vi "Topo & GridSpectr_DriftCorrection_v11.vi"(6 "Internal use":string, 7 "Grid param":T1 {"height (m)" format="%#_6p"; "width (m)" format="%#_6p"; "center Y (m)" format="%#_6p"; "center X (m)" format="%#_6p"}, 8 "Error in (no error)":errorcluster, 9 "Points Y/Index Y":i32, 10 "Points X/Index X":i32, 11 "Method":enum16{"init", "run", "end"}(ring)=enum."end") -> (0 "Error out":errorcluster)   [LabVIEW 2014]
doc: "Example of a measurement VI to be used in the \"Experiments on a Grid\" tool as external VI.\n\nThis example measure the topography and spectroscopy data. The spectroscopy measurements are taken on a subgrid. The data are saved to a sxm and a binary file.\n\n- Nanonis Programming Interface -"
uses:
  <userlib>/Nanonis Prog Interface V5/Scan/Grid/GridPatternGet.vi
  <userlib>/Nanonis Prog Interface V5/Nanonis Prog Interface.lvlib
panel:
  in  "Lockin ON/OFF":bool
  in  "Correct Drift":bool
  in  "Email when finished":string="cornelius.krull@monash.edu"
  in  "STS z offset":dbl=1.15e-09 format="%#_6p"
  out "ETA":timestamp
  out "remaining":dbl format="%<%H:%M:%S>t"
  out "Progress":u8(slide) scale=0.0..100.0 scale format="%#.1g"
  out "total Points":i32
  in  "preSTS delay [ms]":u32=3
  in  "STS Bias":dbl=0.005 format="%#_6p"
  in  "Move Bias":dbl=-0.01 format="%#_6p"
  in  "Move Current":dbl=1.5e-11 format="%#_6p"
  in  "Imaging Bias":dbl=-0.01 format="%#_6p"
  in  "max applied Drift Correction":i32=20 min=1 max=100 step=1 format="%.0p"
  in  "Correlate":u16(ring) items=["first Frame", "successive Frames"]
  out "Topo Images taken":i32=14
  in  "Increment":i32=40
  in  "Threshold":i32=2 min=1 step=1
  in  "tip Speed (m/s)":sgl=1e-08 format="%.2p"
  out "X drift":i32
  out "Y drift":i32
  out "Last Drift detected":i32=40
  in  "MaxImagesBack":i32=40
  in  "Channel index (0-23)":u8=14
  in  "File name":string="single_mol_shortSTS"
  in  "STS Current":dbl=1.15e-09 format="%#_6p"
  in  "Imaging Current":dbl=1.5e-11 format="%#_6p"
  in  "zdrift \nDuration (s)":dbl
  in  "Correct z drift":bool
  out "Status":string="finishing"
  in  "Drift correction Pixels":i32=256 caption="Topo Pixels"
  out "Y Offset":dbl format="%#_6p"
  out "X Offset":dbl format="%#_6p"
  out "Points taken":dbl=14.0
  in  "Drift Correction every":i32=40
  in  "Y subgrid spacing":u16=1
  in  "X subgrid spacing":u16=1
  # "GRID points"
  # "Increase this if no Drift was detected for \na certain number of images"
  # "%"
  # "time (HH:MM:SS)"
  # "images back"
  # "% of image size"
  # "RUN smart tilt before starting the GRID"
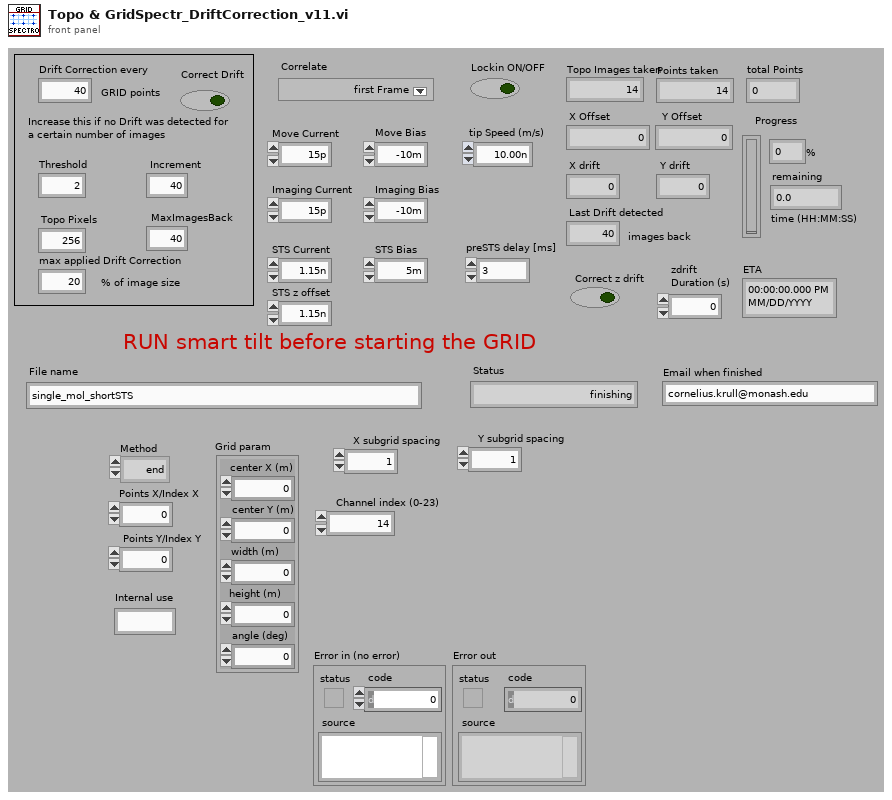
[diagram p1: front panel]
types:
  T1 = cluster{"center X (m)":sgl, "center Y (m)":sgl, "width (m)":sgl, "height (m)":sgl, "angle (deg)":sgl}
  T2 = cluster{"Drift correction Pixels":i32, "Imaging Current":dbl, "STS Current":dbl, "MaxImagesBack":i32, "tip Speed (m/s)":sgl, "Threshold":i32, "Increment":i32, "Correlate":u16, "max applied Drift Correction":i32, "Imaging Bias":dbl, "Move Current":dbl, "Move Bias":dbl, "STS Bias":dbl, "preSTS delay [ms]":u32, "STS z offset":dbl, "Correct Drift":bool, "Lockin ON/OFF":bool}
  T3 = cluster{"center X":sgl, "center Y":sgl, "angle":sgl, "width":sgl, "height":sgl, "# pixels":i32, "# lines":i32}
  T4 = cluster{"Name":string, "Calibration":sgl, "Offset":sgl, "Channel index":i32}[]
  T5 = cluster{"up/down":bool, "time/line":sgl, "start time":timestamp, "end time":timestamp}
  T6 = cluster{"Z averaging time (s)":sgl, "Z offset (m)":sgl, "Initial settling time (s)":sgl}
  T7 = cluster{"Max. slew rate (V/s)":sgl, "Settling time (s)":sgl, "Integration time (s)":sgl}
  T8 = cluster{"End settling time (s)":sgl, "Z control time (s)":sgl}
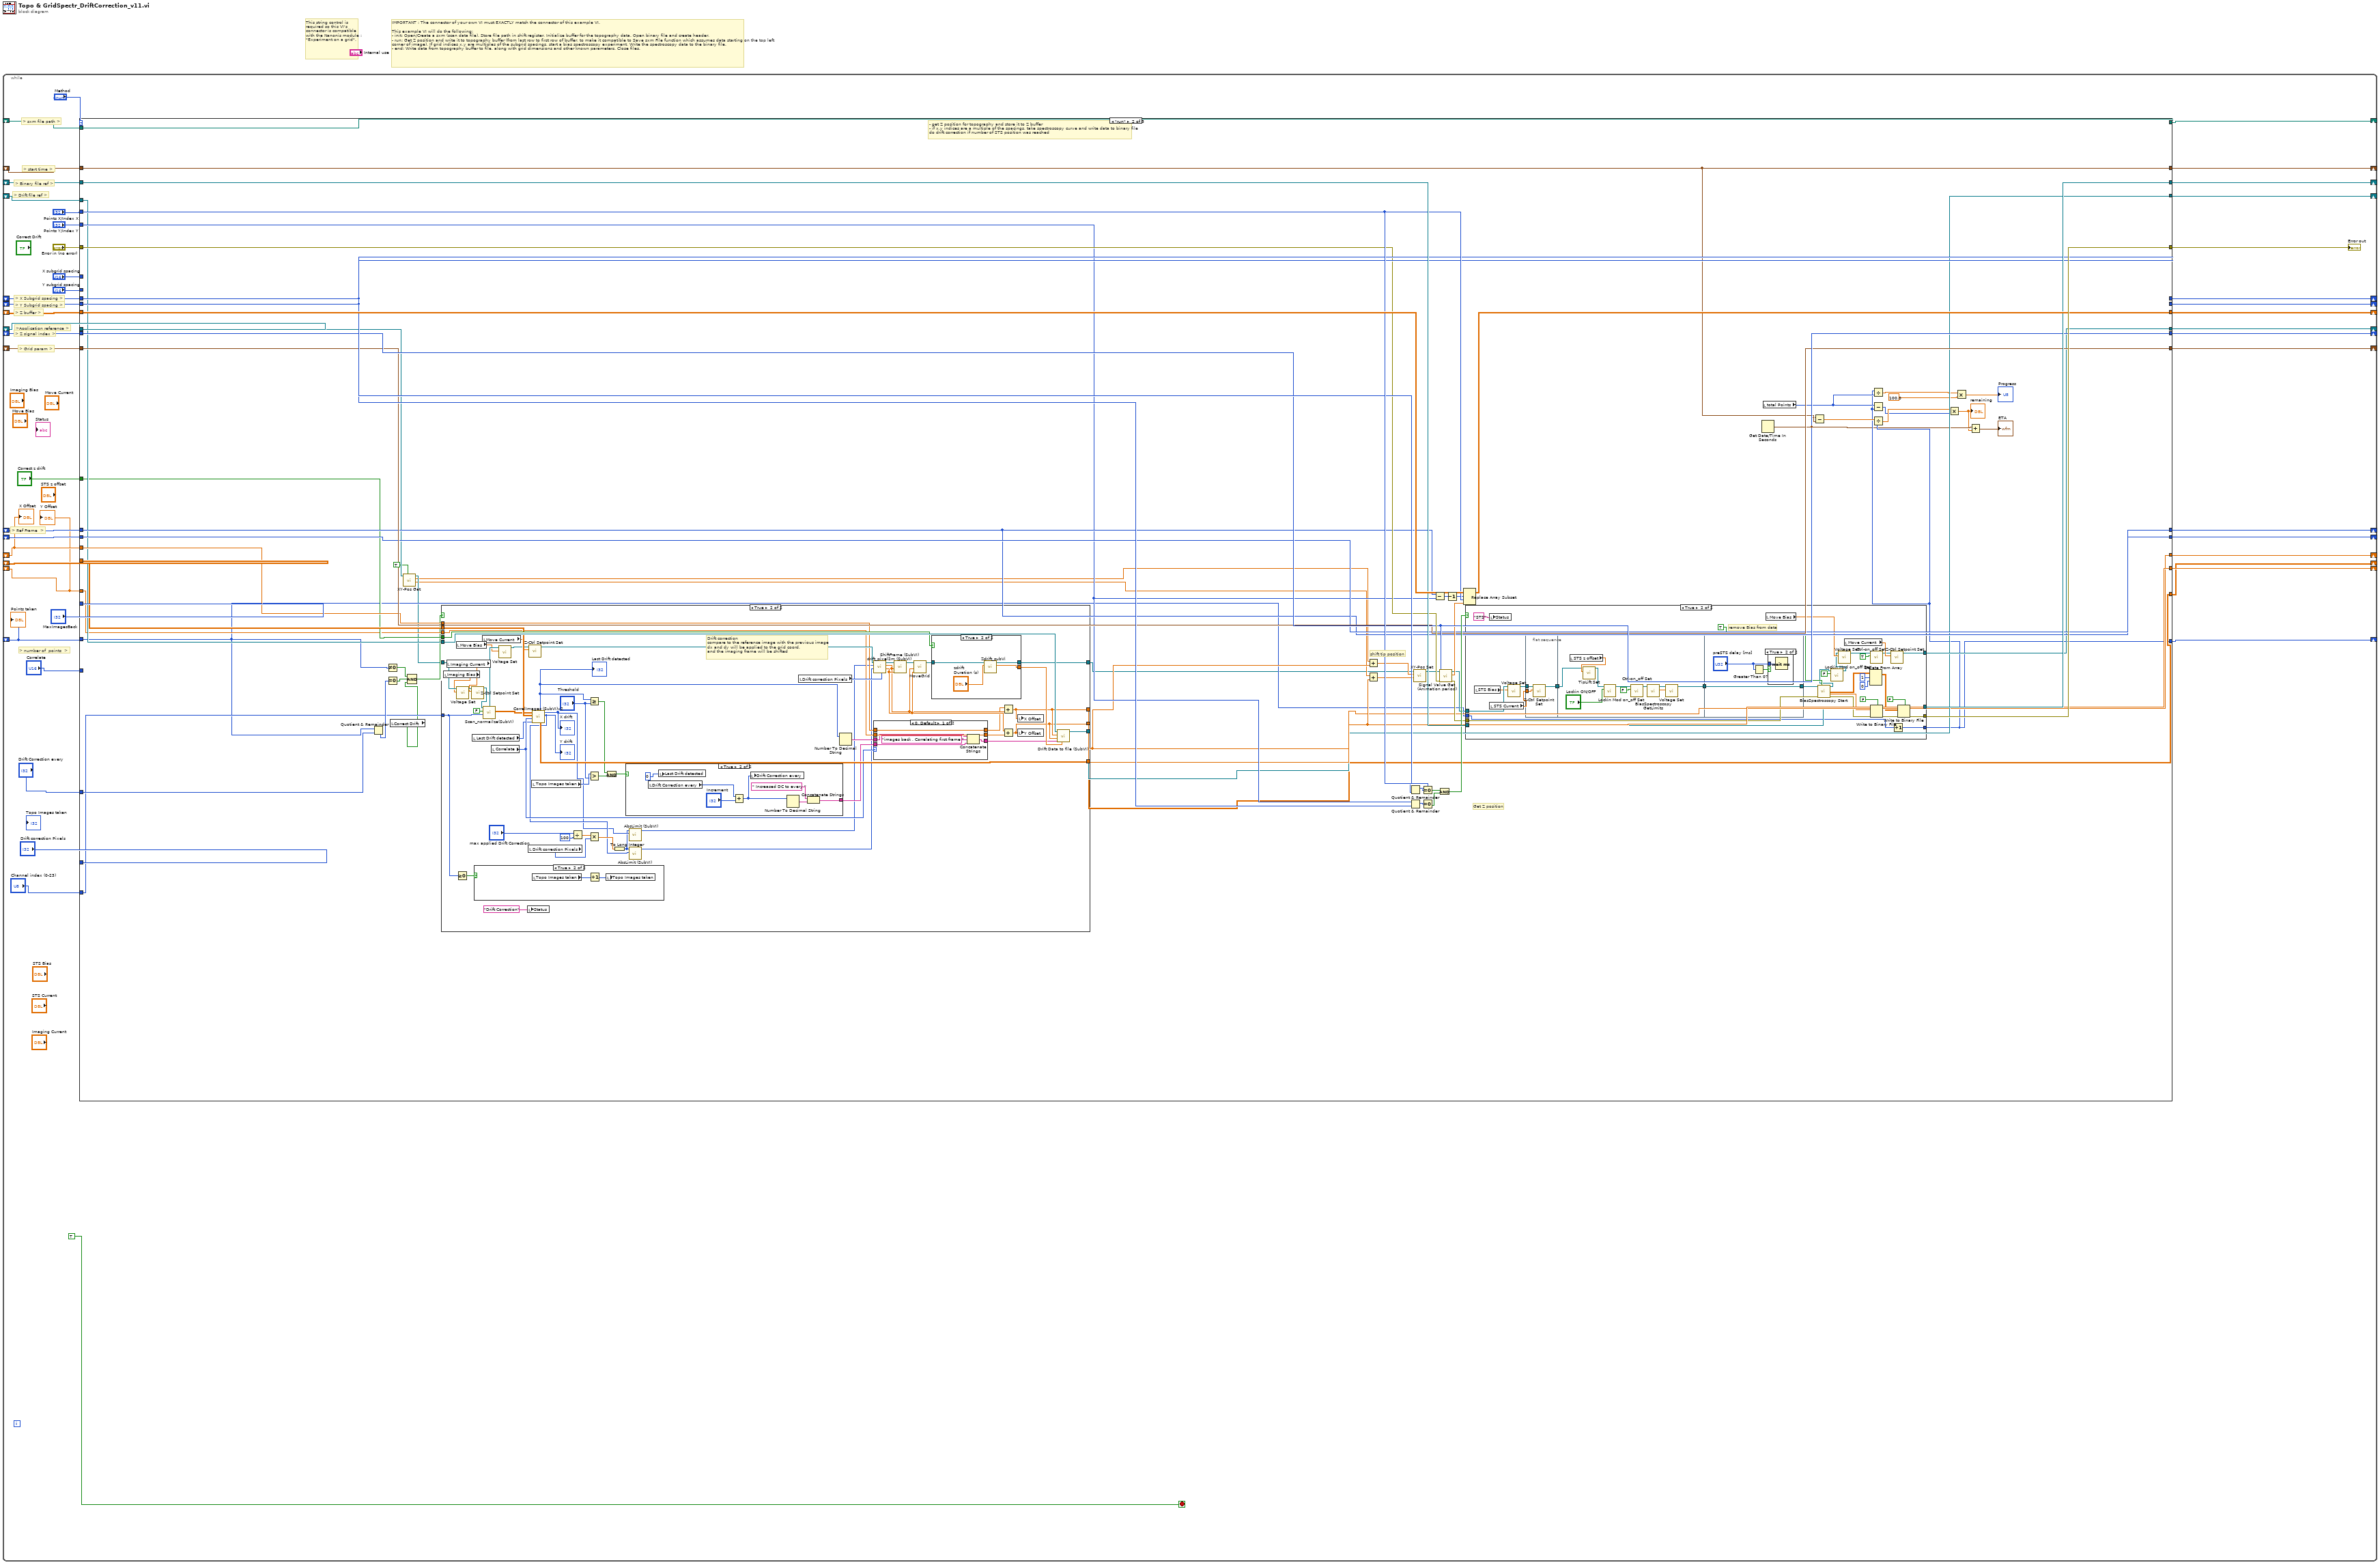
[diagram p0: block diagram]
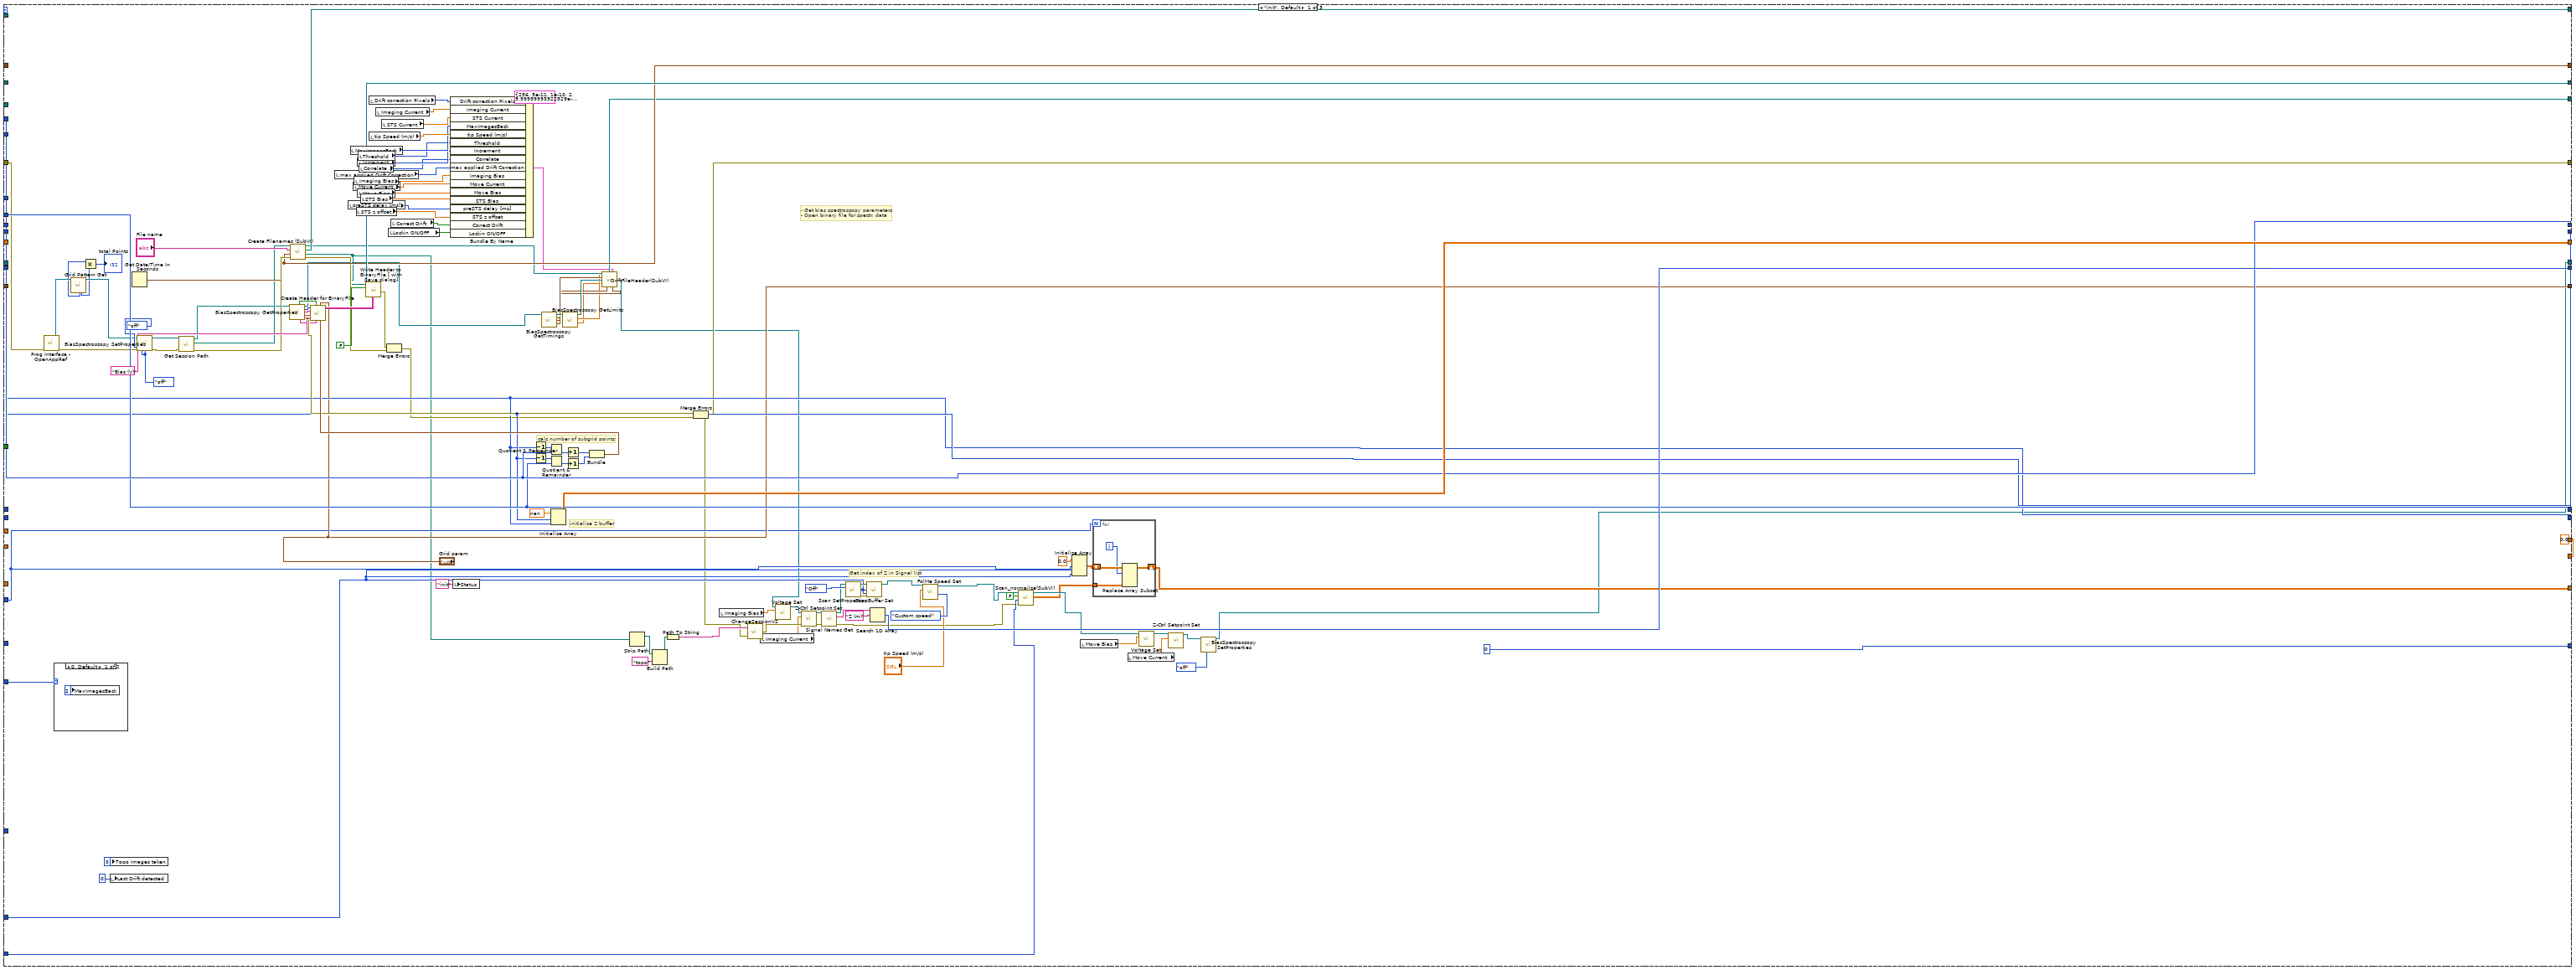
[diagram p2: hidden frame]
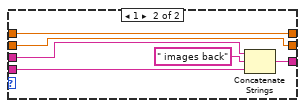
[diagram p5: hidden frame]
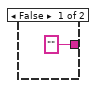
[diagram p7: hidden frame]
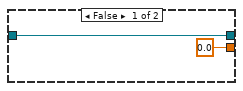
[diagram p8: hidden frame]
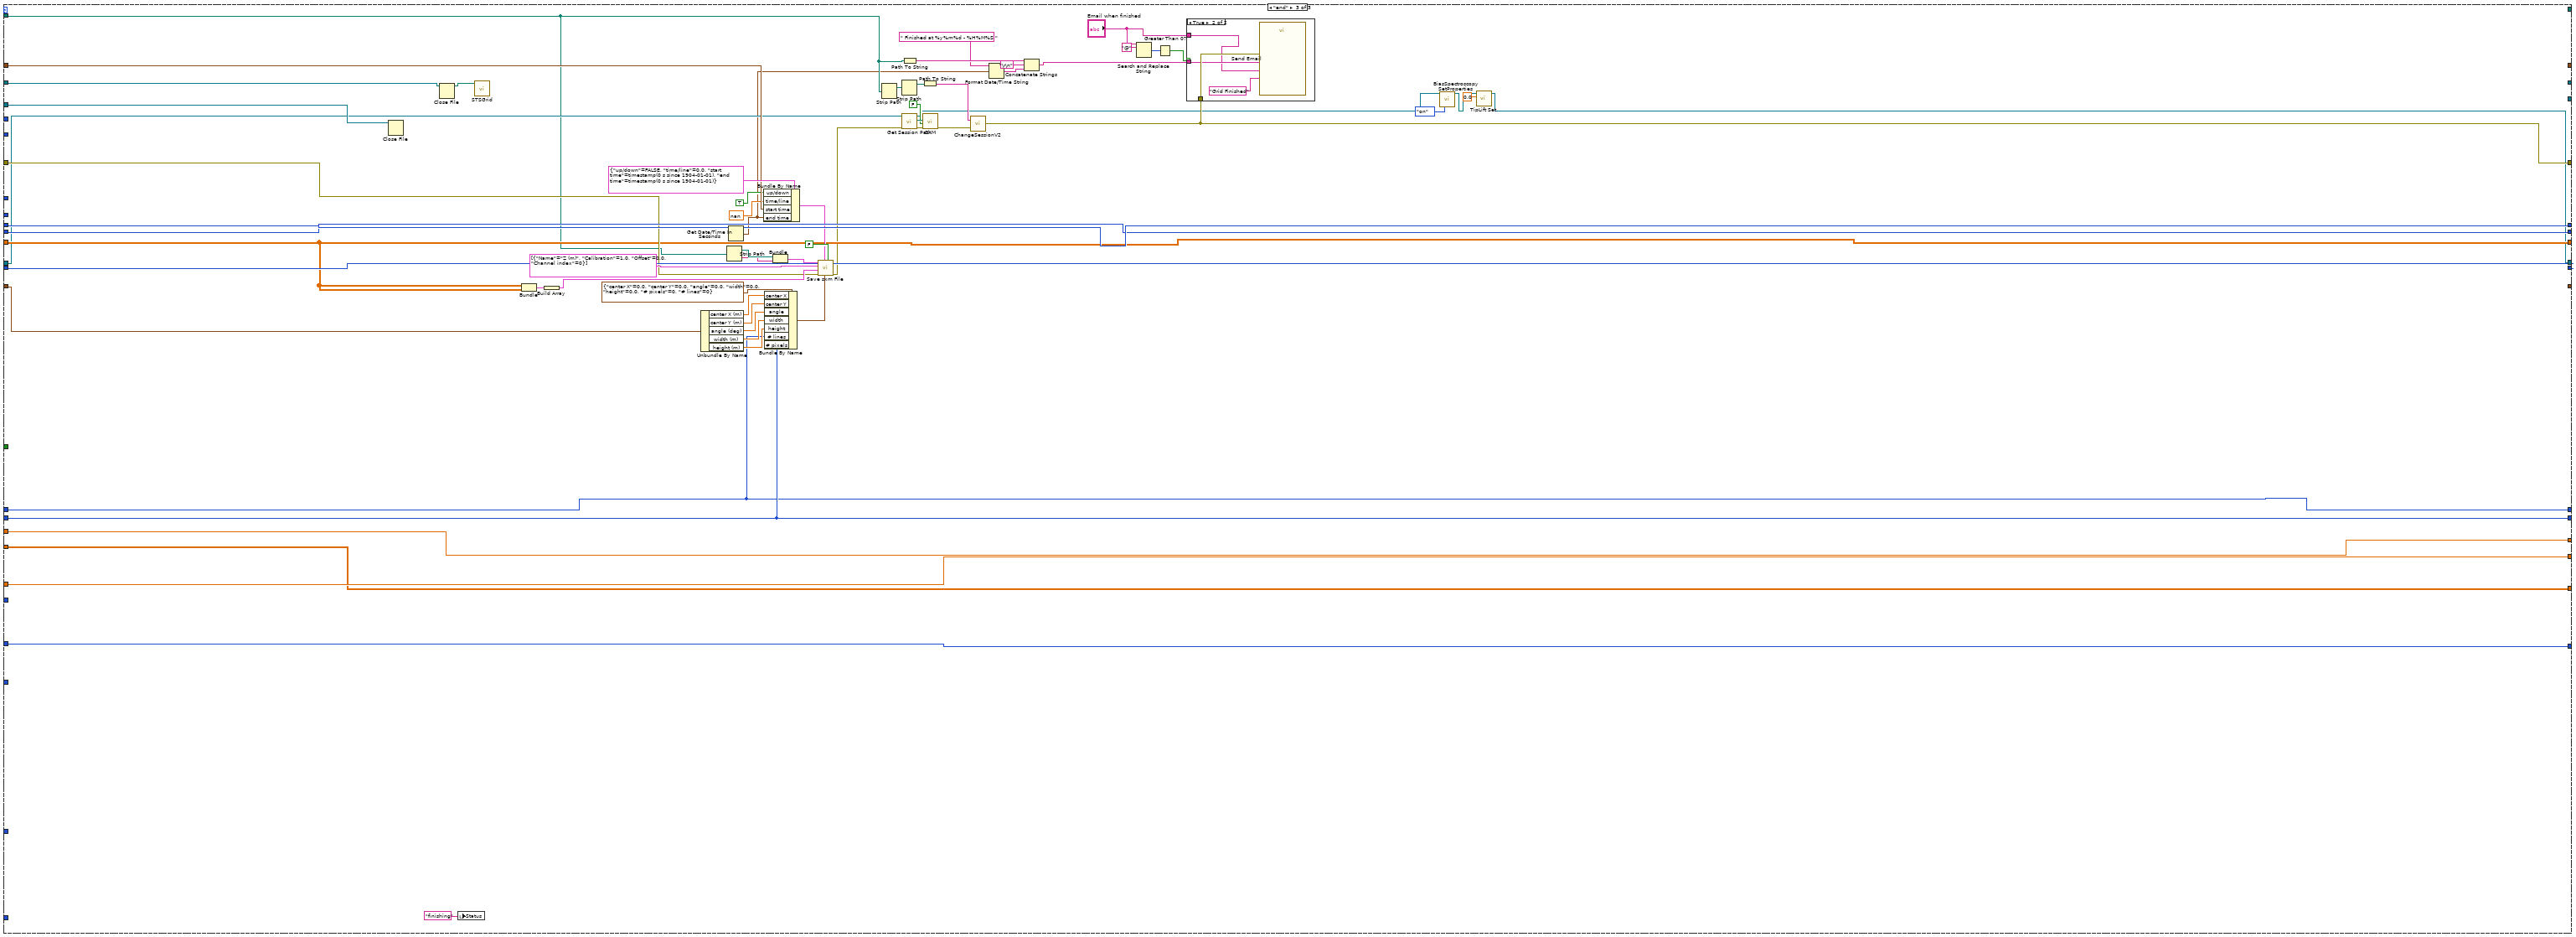
[diagram p11: hidden frame]
diagram:
  # "This string control is required so this VI's connector is compatible with the Nanonis module : \"Experiment on a grid\"."
  # "IMPORTANT : The connector of your own VI must EXACTLY match the connector of this example VI.\n\nThis example VI will do the following:\n- init: Open/Create a sxm (scan data file). Store file path in shift register. Initialize buffer for the topography data. Open binary file and create header.\n- run: Get Z position and write it to topography buffer (from last row to first row of buffer, to make it compatible to Save sxm File function which assumes data starting on the top left corner of image). If grid indices x,y are multiples of the subgrid spacings, start a bias spectroscopy experiment. Write the spectroscopy data to the binary file.\n- end: Write data from topography buffer to file, along with grid dimensions and other known parameters. Close files."
  n1 = while {
    shift-right: [w21] -> _
    shift-left: _ -> [w44]
    shift-right: [w39] -> _
    shift-left: _ -> [w38]
    shift-right: [w36] -> _
    shift-left: _ -> [w37]
    shift-right: [w35] -> _
    shift-left: _ -> [w34]
    shift-right: [w28] -> _
    shift-left: _ -> [w30]
    shift-right: [w29] -> _
    shift-left: _ -> [w31]
    shift-right: [w27] -> _
    shift-left: _ -> [w26]
    shift-right: [w25] -> _
    shift-left: _ -> [w24]
    shift-right: [w23] -> _
    shift-left: _ -> [w22]
    shift-right: [w20] -> _
    shift-left: _ -> [w19]
    shift-right: [w18] -> _
    shift-left: _ -> [w17]
    shift-right: [w16] -> _
    shift-left: _ -> [w9]
    shift-right: [w15] -> _
    shift-left: _ -> [w8]
    shift-right: [w14] -> _
    shift-left: _ -> [w11]
    shift-right: [w13] -> _
    shift-left: _ -> [w10]
    shift-right: [w6] -> _
    shift-left: _ -> [w5]
    stop <- TRUE stop-if-true
    # "> Drift file ref >"
    # "> number of  points  >"
    # "> Ref Frame  >"
    # "> Grid param >"
    # "> start time >"
    # ">Application reference >"
    # "> Y Subgrid spacing >"
    # "> X Subgrid spacing >"
    # "> Z signal index >"
    # "> Binary file ref >"
    # "> Z buffer >"
    # "> sxm file path >"
    n2 = case shown="\"run\"" "Method" {
      tunnel: [w127 w234 _] -> w21
      tunnel: w44 -> [_ w234 w393]
      tunnel: "Error in (no error)" -> [w129 w220 w424]
      tunnel: [w106 w233 w394] -> w42
      tunnel: "Points X/Index X" -> [w141 w228 _]
      tunnel: "Points Y/Index Y" -> [w142 w213 _]
      tunnel: [w165 w231 w413] -> w39
      tunnel: w38 -> [_ w232 w413]
      tunnel: w37 -> [_ w230 w406]
      tunnel: [w157 w229 _] -> w36
      tunnel: [w155 w218 w438] -> w35
      tunnel: w34 -> [_ w218 w438]
      tunnel: "X subgrid spacing" -> [w154 _ _]
      tunnel: "Y subgrid spacing" -> [w153 _ _]
      tunnel: w31 -> [_ w222 w437]
      tunnel: w30 -> [_ w221 w436]
      tunnel: [w154 w222 w437] -> w29
      tunnel: [w153 w221 w436] -> w28
      tunnel: [w84 w206 w379] -> w27
      tunnel: w26 -> [_ w189 w399]
      tunnel: ["Grid param" w216 _] -> w25
      tunnel: w24 -> [_ w216 w423]
      tunnel: [w126 w179 _] -> w23
      tunnel: w22 -> [_ w179 w431]
      tunnel: [w142 w214 w414] -> w20
      tunnel: w19 -> [_ w214 w414]
      tunnel: [w141 w215 w415] -> w18
      tunnel: w17 -> [_ w215 w415]
      tunnel: [w138 w196 w412] -> w16
      tunnel: [w138 w201 w410] -> w15
      tunnel: [w122 w195 w407] -> w14
      tunnel: [0 w177 w411] -> w13
      tunnel: w10 -> [_ w192 w411]
      tunnel: "Drift Correction every" -> [_ w209 _]
      tunnel: w11 -> [_ w200 w407]
      tunnel: w9 -> [_ w207 w412]
      tunnel: w8 -> [_ w193 w410]
      tunnel: "Drift correction Pixels" -> [w121 _ _]
      tunnel: [w79 w198 _] -> w6
      tunnel: w5 -> [_ w199 w408]
      tunnel: "Correct z drift" -> [_ w197 _]
      tunnel: "Channel index (0-23)" -> [w52 w194 _]
      tunnel: "MaxImagesBack" -> [w120 _ _]
      tunnel: "Correlate" -> [w98 _ _]
      frame "init", Default {
        w81 = enum16{"no change", "on", "off"}."off" ("Save dialog")
        w138 = 0.0
        # "- Get bias spectroscopy parameters\n- Open binary file for spectr. data"
        # "initialize Z buffer"
        # "calc number of subgrid points"
        # "Get index of Z in Signal list"
        n3 = call <userlib>:"Prog Interface - OpenAppRef.vi"("Error in (no error)"=w129) -> ("Error out"=w104:errorcluster, "Application reference"=w89:refnum<vi>)  [unwired: 5 in]
        n4 = case shown="0, Default" w98 {
          frame 0, Default {
            n5 = local write "MaxImagesBack"(2 ("StepsBack")) -> ()
          }
          frame 1 {
          }
        }
        n6 = call-poly <userlib>:"Grid Pattern Get.vi"("Application ref in"=w89) -> ("Points Y"=w86:i32, "Points X"=w87:i32, "Application ref out"=w88:refnum<vi>)  [unwired: 10 in, 6 out]
        n7 = Multiply(x=w86, y=w87) -> (x*y=→"total Points":i32)
        n8 = local write "Topo Images taken"(0 ("Images taken")) -> ()
        n9 = local write "Last Drift detected"(0 ("Last Drift detected")) -> ()
        n10 = Get Date/Time In Seconds() -> (seconds since 1Jan1904=w126:timestamp)
        n11 = call <userlib>:"BiasSpectroscopy SetProperties.vi"("Application ref in"=w88, "Autosave (no change)"=enum16{"no change", "on", "off"}."off", "Error in (no error)"=w104, "Z-Controller hold (no change)"=w81, "Save dialog"=w81) -> ("Application ref out"=w101:refnum<vi>, "Error out"=w100:errorcluster)  [unwired: 9 in]
        n12 = call <userlib>:"Get Session Path.vi"("error in (no error)"=w100, "Application ref in"=w101) -> ("error out"=w128:errorcluster, "Session path"=w112:path, "Application ref out"=w102:refnum<vi>)  [unwired: 7 in]
        n13 = call <userlib>:"BiasSpectroscopy GetProperties.vi"("Application ref in"=w102) -> ("Backward sweep"=w161:bool, "Application ref out"=w115:refnum<vi>, "Number of points"=w144:i32, "Channels"=w143:string[], "Parameters"=w159:string[], "Fixed parameters"=w146:string[], "Error out"=w158:errorcluster)  [unwired: 6 in, 2 out]
        n14 = call "Create Filenames (SubVI).vi"("error in (no error)"=w128, "seconds since 1Jan1904"=w126, "File name"="File name", "Session path"=w112) -> ("error out"=w116:errorcluster, "binFilePath"=w108:path, "topoFilePath"=w127:path, "Drift File out"=w80:refnum<file>)  [unwired: 4 in]
        n15 = local read "max applied Drift Correction"() -> (w60:i32)
        n16 = local read "preSTS delay [ms]"() -> (w55:u32)
        n17 = local read "MaxImagesBack"() -> (w64:i32)
        n18 = local read "Move Current"() -> (w58:dbl)
        n19 = local read "Imaging Bias"() -> (w59:dbl)
        n20 = local read "STS z offset"() -> (w54:dbl)
        n21 = local read "Increment"() -> (w62:i32)
        n22 = local read "Move Bias"() -> (w57:dbl)
        n23 = local read "Threshold"() -> (w63:i32)
        n24 = local read "Correlate"() -> (w61:u16)
        n25 = local read "STS Bias"() -> (w56:dbl)
        n26 = local read "Drift correction Pixels"() -> (w69:i32)
        n27 = local read "tip Speed (m/s)"() -> (w66:sgl)
        n28 = local read "Imaging Current"() -> (w68:dbl)
        n29 = local read "STS Current"() -> (w67:dbl)
        n30 = local read "Lockin ON/OFF"() -> (w65:bool)
        n31 = local read "Correct Drift"() -> (w53:bool)
        n32 = Bundle By Name(cluster=T2 {"Drift correction Pixels"=256, "Imaging Current"=5e-11, "STS Current"=1e-10, "MaxImagesBack"=2, "tip Speed (m/s)"=1e-08, "Threshold"=2, "Increment"=64, "Correlate"=0, "max applied Drift Correction"=20, "Imaging Bias"=-0.02, "Move Current"=1.5e-11, "Move Bias"=-0.02, "STS Bias"=0.1, "preSTS delay [ms]"=1000, "STS z offset"=-1.7e-10, "Correct Drift"=TRUE, "Lockin ON/OFF"=TRUE} ("Drift Correction"), "Drift correction Pixels"=w69, "Imaging Current"=w68, "STS Current"=w67, "MaxImagesBack"=w64, "tip Speed (m/s)"=w66, "Threshold"=w63, "Increment"=w62, "Correlate"=w61, "max applied Drift Correction"=w60, "Imaging Bias"=w59, "Move Current"=w58, "Move Bias"=w57, "STS Bias"=w56, "preSTS delay [ms]"=w55, "STS z offset"=w54, "Correct Drift"=w53, "Lockin ON/OFF"=w65) -> (w71:T2)
        n33 = local write "Status"("init" ("Status")) -> ()
        n34 = Decrement(x=w141) -> (x-1=w152:i32)
        n35 = Decrement(x=w142) -> (x-1=w151:i32)
        n36 = call <userlib>:"BiasSpectroscopy GetTimings.vi"("Application ref in"=w115) -> ("Application ref out"=w119:refnum<vi>, "Initialization"=w74:T6, "Sweep Timing"=w75:T7, "End of Sweep"=w76:T8)  [unwired: 10 in, 1 out]
        n37 = Quotient & Remainder(x=w152, y=w154) -> (floor(x/y)=w150:i32)  [unwired: 1 out]
        n38 = Quotient & Remainder(x=w151, y=w153) -> (floor(x/y)=w149:i32)  [unwired: 1 out]
        n39 = Initialize Array(sgl nan ("element"), w142, w141) -> (w165:sgl[][])
        n40 = call <userlib>:"BiasSpectroscopy GetLimits.vi"("Application ref in"=w119) -> ("End value (V)"=w72:sgl, "Start value (V)"=w73:sgl, "Application ref out"=w78:refnum<vi>)  [unwired: 5 in, 1 out]
        n41 = Increment(x=w150) -> (x+1=w148:i32)
        n42 = Increment(x=w149) -> (x+1=w147:i32)
        n43 = Bundle(w148, w147) -> (w160:cluster{i32, i32})  [unwired: 1 in]
        n44 = call <userlib>:"Create Header for BinaryFile.vi"("Grid points"=w160, "Grid param"="Grid param", "Fixed parameters"=w146, "Backward sweep"=w161, "Sweep signal"="Bias (V)" ("Sweep Signal"), "Parameters"=w159, "Channels"=w143, "Points per sweep"=w144) -> ("Header (fixed attributes)"=w163:string[][])  [unwired: 3 in]
        n45 = call <userlib>:"Write Header to BinaryFile [ with Save dialog].vi"("Fixed Attributes"=w163, "Show Dialog? (T)"=FALSE, "Filename"=w108) -> ("Error out"=w117:errorcluster, "File ref"=w157:refnum<file>)  [unwired: 5 in, 2 out]
        n46 = Merge Errors(w117, w116) -> (w118:errorcluster)
        n47 = call "DriftFileHeader(SubVI).vi"("Start value (V)"=w73, "Byte Stream File in"=w80, "Drift Correction"=w71, "End of Sweep"=w76, "Application ref in"=w78, "End value (V)"=w72, "Sweep Timing"=w75, "Initialization"=w74) -> ("Byte Stream File out"=w79:refnum<file>, "Application ref out"=w77:refnum<vi>)  [unwired: 6 in]
        n48 = Strip Path(path=w108) -> (stripped path=w111:path)  [unwired: 1 out]
        n49 = Build Path(base path=w111, name or relative path="topo") -> (appended path=w109:path)
        n50 = Path To String(path=w109) -> (string=w107:string)
        n51 = Merge Errors(w158, w118) -> (w106:errorcluster)
        n52 = local read "Imaging Bias"() -> (w91:dbl)
        n53 = call "ChangeSessionV2.vi"("error in (no error)"=w106, "Session"=w107) -> ("error out"=w105:errorcluster)
        n54 = local read "Imaging Current"() -> (w90:dbl)
        n55 = call <userlib>:"Voltage Set.vi"("Bias (V)"=w91, "Application ref in"=w77) -> ("Application ref out"=w94:refnum<vi>)  [unwired: 8 in, 1 out]
        n56 = call <userlib>:"Z-Ctrl Setpoint Set.vi"("error in (no error)"=w105, "Z Controller setpoint"=w90, "Application ref in"=w94) -> ("error out"=w130:errorcluster, "Application ref out"=w131:refnum<vi>)  [unwired: 7 in]
        n57 = call <userlib>:"Signal Names Get.vi"("error in (no error)"=w130, "Application ref in"=w131) -> ("error out"=w49:errorcluster, "Signals Names"=w145:string[], "Application ref out"=w134:refnum<vi>)  [unwired: 5 in]
        n58 = call <userlib>:"Scan SetProperties.vi"("Application ref in"=w134, "Continuous scan"=enum16{"No change", "On", "Off"}."Off") -> ("Application ref out"=w136:refnum<vi>, "Error out"=w135:errorcluster)  [unwired: 12 in]
        n59 = call <userlib>:"ScanBuffer Set.vi"("Application ref in"=w136, "Pixels"=w121, "Lines"=w121, "error in (no error)"=w135) -> ("Application ref out"=w96:refnum<vi>)  [unwired: 10 in, 1 out]
        n60 = Search 1D Array(1D array=w145, element="Z (m)") -> (index of element=w155:i32)  [unwired: 1 in]
        n61 = call <userlib>:"FolMe Speed Set.vi"("Speed Setting (Custom)"=enum32{"Scan speed", "Custom speed"}."Custom speed", "Speed (m/s)"="tip Speed (m/s)", "Application ref in"=w96) -> ("Application ref out"=w51:refnum<vi>)  [unwired: 5 in, 1 out]
        n62 = call "Scan_normailze(SubVI).vi"("error in (no error)"=w49, "Channel index (0-23)"=w52, "Normalization"=FALSE ("Boolean"), "Application in"=w51) -> ("Array"=w48:dbl[][], "Application out"=w50:refnum<vi>)  [unwired: 5 in, 1 out]
        n63 = Initialize Array(0.0 ("element"), w120, w121, w121) -> (w123:dbl[][][])
        n64 = local read "Move Bias"() -> (w93:dbl)
        n65 = for {
          N: w120 -> [_]
          tunnel: w48 -> [w169]
          shift-right: [w168] -> w122
          shift-left: w123 -> [w170]
          i -> [w167]
          n66 = Replace Array Subset(array=w170, new element=w169, index (dim 0)=w167) -> (w168:dbl[][][])  [unwired: 2 in]
        }
        n67 = local read "Move Current"() -> (w92:dbl)
        n68 = call <userlib>:"Voltage Set.vi"("Bias (V)"=w93, "Application ref in"=w50) -> ("Application ref out"=w95:refnum<vi>)  [unwired: 8 in, 1 out]
        n69 = call <userlib>:"Z-Ctrl Setpoint Set.vi"("Z Controller setpoint"=w92, "Application ref in"=w95) -> ("Application ref out"=w83:refnum<vi>)  [unwired: 8 in, 1 out]
        n70 = call <userlib>:"BiasSpectroscopy SetProperties.vi"("Application ref in"=w83, "Z-Controller hold (no change)"=enum16{"no change", "on", "off"}."off") -> ("Application ref out"=w84:refnum<vi>)  [unwired: 12 in, 1 out]
      }
      frame "run" {
        # "shift tip position"
        # "Get Z position"
        # "- get Z position for topography and store it to Z buffer\n- if x,y indices are a multiple of the spacings, take spectroscopy curve and write data to binary file\ndo drift correction if number of STS position was reached"
        n71 = Quotient & Remainder(x=w192, y=w209) -> (x-y*floor(x/y)=w210:i32)  [unwired: 1 out]
        n72 = Not Equal To 0?(x=w192) -> (x != 0?=w190:bool)
        n73 = Equal To 0?(x=w210) -> (x = 0?=w208:bool)
        n74 = local read "Correct Drift"() -> (w171:bool)
        n75 = call <userlib>:"XY-Pos Get.vi"("Wait for newest data (F=False)"=TRUE, "Application ref in"=w189) -> ("Y (m)"=w185:sgl, "X (m)"=w186:sgl, "Application ref out"=w188:refnum<vi>)  [unwired: 5 in, 1 out]
        n76 = Compound Arithmetic op=AND(w190, w208, w171) -> (w191:bool)
        n77 = case shown="True" w191 {
          tunnel: w188 -> [w239 w248]
          tunnel: [w239 w290] -> w184
          tunnel: w200 -> [w236 w285]
          tunnel: [w238 w288] -> w196
          tunnel: [w237 w287] -> w201
          tunnel: w207 -> [w238 w264]
          tunnel: w193 -> [w237 w262]
          tunnel: [w236 w281] -> w195
          tunnel: w199 -> [w235 w293]
          tunnel: [w235 w292] -> w198
          tunnel: w197 -> [_ w289]
          tunnel: w194 -> [_ w268]
          frame False {
          }
          frame True {
            # "Drift correction \ncompare to the reference image with the previous image \ndx and dy will be applied to the grid coord, \nand the imaging frame will be shifted"
            n78 = local read "Imaging Bias"() -> (w246:dbl)
            n79 = local read "Imaging Current"() -> (w245:dbl)
            n80 = local read "Move Bias"() -> (w242:dbl)
            n81 = Greater Or Equal To 0?(x=w268) -> (x >= 0?=w267:bool)
            n82 = call <userlib>:"Voltage Set.vi"("Bias (V)"=w246, "Application ref in"=w248) -> ("Application ref out"=w247:refnum<vi>)  [unwired: 8 in, 1 out]
            n83 = call <userlib>:"Z-Ctrl Setpoint Set.vi"("Z Controller setpoint"=w245, "Application ref in"=w247) -> ("Application ref out"=w286:refnum<vi>)  [unwired: 8 in, 1 out]
            n84 = local read "Last Drift detected"() -> (w259:i32)
            n85 = case shown="True" w267 {
              frame False {
              }
              frame True {
                n86 = local read "Topo Images taken"() -> (w308:i32)
                n87 = Increment(x=w308) -> (x+1=w307:i32)
                n88 = local write "Topo Images taken"(w307) -> ()
              }
            }
            n89 = local read "Move Current"() -> (w241:dbl)
            n90 = call "Scan_normailze(SubVI).vi"("Channel index (0-23)"=w268, "Normalization"=FALSE ("Boolean"), "Application in"=w286) -> ("Array"=w282:dbl[][], "Application out"=w243:refnum<vi>)  [unwired: 6 in, 1 out]
            n91 = local read "Correlate"() -> (w265:u16)
            n92 = call <userlib>:"Voltage Set.vi"("Bias (V)"=w242, "Application ref in"=w243) -> ("Application ref out"=w244:refnum<vi>)  [unwired: 8 in, 1 out]
            n93 = local write "Status"("Drift Correction" ("Status")) -> ()
            n94 = local read "Drift correction Pixels"() -> (w256:i32)
            n95 = call <userlib>:"Z-Ctrl Setpoint Set.vi"("Z Controller setpoint"=w241, "Application ref in"=w244) -> ("Application ref out"=w277:refnum<vi>)  [unwired: 8 in, 1 out]
            n96 = local read "Topo Images taken"() -> (w270:i32)
            n97 = call "CorrelImages (SubVI)v2.vi"("last drift detected"=w259, "Correlate"=w265, "Ref Array"=w285, "New Image"=w282) -> ("Y drift"=w253:i32, "X drift"=w250:i32, "Ref Array out"=w281:dbl[][][], "Queue Steps"=w266:i32)  [unwired: 4 in]
            "X drift" <- w250
            "Y drift" <- w253
            "Last Drift detected" <- w266
            n98 = Divide(x="max applied Drift Correction", y=100) -> (x/y=w255:dbl)
            n99 = Greater Or Equal?(x=w266, y="Threshold") -> (x >= y?=w272:bool)
            n100 = Greater?(x=w270, y="Threshold") -> (0:w269:bool)
            n101 = Multiply(x=w255, y=w256) -> (x*y=w257:dbl)
            n102 = And(x=w272, y=w269) -> (x .and. y?=w271:bool)
            n103 = To Long Integer(number=w257) -> (32bit integer=w249:i32)
            n104 = case shown="True" w271 {
              tunnel: ["" w312] -> w273
              frame False {
              }
              frame True {
                n105 = local read "Drift Correction every"() -> (w311:i32)
                n106 = local write "Last Drift detected"(0 ("Last Drift detected")) -> ()
                n107 = Add(x=w311, y="Increment") -> (x+y=w315:i32)
                n108 = local write "Drift Correction every"(w315) -> ()
                n109 = Number To Decimal String(number=w315) -> (decimal integer string=w314:string)  [unwired: 1 in]
                n110 = Concatenate Strings(" Increased DC to every " ("string"), w314) -> (w312:string)
              }
            }
            n111 = call "AbsLimit (SubVI).vi"("in"=w250, "Abslimt"=w249) -> ("Numeric out"=w252:i32)  [unwired: 9 in]
            n112 = call "AbsLimit (SubVI).vi"("in"=w253, "Abslimt"=w249) -> ("Numeric out"=w251:i32)  [unwired: 9 in]
            n113 = local read "Drift correction Pixels"() -> (w278:i32)
            n114 = Number To Decimal String(number=w266) -> (decimal integer string=w284:string)  [unwired: 1 in]
            n115 = call "drift_pixel2m (SubVI).vi"("Application in"=w277, "X drift"=w252, "Y drift"=w251, "Drift correction Pixels"=w278) -> ("Application out"=w276:refnum<vi>, "x drift"=w274:sgl, "y drift"=w275:sgl)  [unwired: 2 in, 1 out]
            n116 = case shown="0, Default" w265 {
              tunnel: w284 -> [w295 w306]
              tunnel: [w300 w305] -> w283
              tunnel: w273 -> [w298 w303]
              tunnel: w264 -> [w296 w302]
              tunnel: [w296 w302] -> w263
              tunnel: w262 -> [w297 w301]
              tunnel: [w297 w301] -> w261
              frame 0, Default {
                n117 = Concatenate Strings(w295, "images back , Correlating first frame " ("string"), w298) -> (w300:string)
              }
              frame 1 {
                n118 = Concatenate Strings(w306, " images back" ("string"), w303) -> (w305:string)
              }
            }
            n119 = call "ShiftFrame (SubVI).vi"("Y shift"=w275, "X shift"=w274, "Application in"=w276) -> ("Application out"=w280:refnum<vi>)  [unwired: 8 in]
            n120 = call "MoveGrid.vi"("y"=w275, "x"=w274, "Application ref in"=w280) -> ("Application ref out"=w279:refnum<vi>)  [unwired: 7 in, 1 out]
            n121 = case shown="True" w289 {
              tunnel: [0.0 ("z drift") w322] -> w291
              tunnel: w279 -> [w317 w321]
              tunnel: [w317 w320] -> w290
              frame False {
              }
              frame True {
                n122 = call "Zdrift_subVi.vi"("Duration"="zdrift \nDuration (s)", "Application in"=w321) -> ("z drift"=w322:dbl, "Application out"=w320:refnum<vi>)  [unwired: 7 in, 1 out]
              }
            }
            n123 = Add(x=w263, y=w274) -> (x+y=w288:dbl)
            n124 = Add(x=w275, y=w261) -> (x+y=w287:dbl)
            n125 = local write "X Offset"(w288) -> ()
            n126 = local write "Y Offset"(w287) -> ()
            n127 = call "Drift Data to file (SubVI).vi"("z drift"=w291, "Comment"=w283, "y Drift"=w287, "X drift"=w288, "Byte Stream File in"=w293) -> ("Byte Stream File out"=w292:refnum<file>)  [unwired: 6 in]
          }
        }
        n128 = Add(x=w186, y=w196) -> (x+y=w203:dbl)
        n129 = Add(x=w185, y=w201) -> (x+y=w202:dbl)
        n130 = Quotient & Remainder(x=w228, y=w222) -> (x-y*floor(x/y)=w227:i32)  [unwired: 1 out]
        n131 = Quotient & Remainder(x=w213, y=w221) -> (x-y*floor(x/y)=w226:i32)  [unwired: 1 out]
        n132 = call <userlib>:"XY-Pos Set.vi"("Y (m)"=w202, "X (m)"=w203, "Application ref in"=w184) -> ("Application ref out"=w204:refnum<vi>)  [unwired: 5 in, 1 out]
        n133 = Equal To 0?(x=w227) -> (x = 0?=w225:bool)
        n134 = Equal To 0?(x=w226) -> (x = 0?=w224:bool)
        n135 = Subtract(x=w214, y=w213) -> (x-y=w212:i32)
        n136 = And(x=w225, y=w224) -> (x .and. y?=w223:bool)
        n137 = call <userlib>:"Signal Value Get (Animation period).vi"("error in (no error)"=w220, "Signal index (0-47)"=w218, "Application ref in"=w204) -> ("error out"=w219:errorcluster, "Signal value"=w217:sgl, "Application ref out"=w205:refnum<vi>)  [unwired: 5 in]
        n138 = Decrement(x=w212) -> (x-1=w211:i32)
        n139 = Replace Array Subset(array=w232, new element=w217, index (row)=w211, index (col)=w228) -> (w231:sgl[][])
        n140 = case shown="True" w223 {
          tunnel: [w325 w346] -> w233
          tunnel: w230 -> [w326 w360]
          tunnel: [w326 w358] -> w229
          tunnel: w219 -> [w325 w357]
          tunnel: w205 -> [w324 w342]
          tunnel: [w324 w337] -> w206
          tunnel: [w323 w344] -> w177
          tunnel: w192 -> [w323 w345]
          frame False {
            # "Point indices aren't multiple of subgrid spacing\n=> no spectroscopy at this point"
          }
          frame True {
            # "remove Bias from data"
            n141 = local read "STS Bias"() -> (w339:dbl)
            n142 = local write "Status"("STS" ("Status")) -> ()
            n143 = local read "STS Current"() -> (w338:dbl)
            n144 = call <userlib>:"Voltage Set.vi"("Bias (V)"=w339, "Application ref in"=w342) -> ("Application ref out"=w341:refnum<vi>)  [unwired: 8 in, 1 out]
            n145 = flat-sequence {
              tunnel: w341 -> [w363]
              tunnel: w338 -> [w361]
              tunnel: [w362] -> w334
              tunnel: w334 -> [w366]
              tunnel: [w364] -> w333
              tunnel: [w376] -> w340
              tunnel: w333 -> [w376]
              frame #0 {
                n146 = call <userlib>:"Z-Ctrl Setpoint Set.vi"("Z Controller setpoint"=w361, "Application ref in"=w363) -> ("Application ref out"=w362:refnum<vi>)  [unwired: 8 in, 1 out]
              }
              frame #1 {
                n147 = local read "STS z offset"() -> (w369:dbl)
                n148 = call <userlib>:"TipLift Set.vi"("TipLift (m)"=w369, "Application ref in"=w366) -> ("Application ref out"=w365:refnum<vi>)  [unwired: 8 in, 1 out]
                n149 = call <userlib>:"Lockin Mod on_off Set.vi"("Lockin ON/OFF"="Lockin ON/OFF", "Application ref in"=w365) -> ("Application ref out"=w368:refnum<vi>)  [unwired: 8 in, 1 out]
                n150 = call <userlib>:"Ctrl-on_off Set.vi"("Z Controller ON/OFF"=FALSE, "Application ref in"=w368) -> ("Application ref out"=w371:refnum<vi>)  [unwired: 8 in, 1 out]
                n151 = call <userlib>:"BiasSpectroscopy GetLimits.vi"("Application ref in"=w371) -> ("Start value (V)"=w370:sgl, "Application ref out"=w372:refnum<vi>)  [unwired: 5 in, 2 out]
                n152 = call <userlib>:"Voltage Set.vi"("Bias (V)"=w370, "Application ref in"=w372) -> ("Application ref out"=w364:refnum<vi>)  [unwired: 8 in, 1 out]
              }
              frame #2 {
                n153 = Greater Than 0?(x="preSTS delay [ms]") -> (x > 0?=w374:bool)
                n154 = case shown="True" w374 {
                  tunnel: "preSTS delay [ms]" -> [_ w377]
                  frame False {
                  }
                  frame True {
                    n155 = Wait (ms)(milliseconds to wait=w377) -> ()  [unwired: 1 out]
                  }
                }
              }
            }
            n156 = local read "Move Bias"() -> (w336:dbl)
            n157 = call <userlib>:"BiasSpectroscopy Start.vi"("Application ref in"=w340, "Get data (F)"=TRUE ("Get Data (F)"), "Error in (no error)"=w357) -> ("Application ref out"=w329:refnum<vi>, "Data"=w356:sgl[][], "Parameters"=w355:sgl[], "Error out"=w348:errorcluster)  [unwired: 8 in, 1 out]
            n158 = call <userlib>:"Lockin Mod on_off Set.vi"("Lockin ON/OFF"=FALSE, "Application ref in"=w329) -> ("Application ref out"=w328:refnum<vi>)  [unwired: 8 in, 1 out]
            n159 = call <userlib>:"Voltage Set.vi"("Bias (V)"=w336, "Application ref in"=w328) -> ("Application ref out"=w331:refnum<vi>)  [unwired: 8 in, 1 out]
            n160 = local read "Move Current"() -> (w335:dbl)
            n161 = Delete From Array(array=w356, length=1, index (row)=0 ("index")) -> (array with subset deleted=w354:sgl[][])  [unwired: 1 in, 1 out]
            n162 = call <userlib>:"Ctrl-on_off Set.vi"("Z Controller ON/OFF"=TRUE, "Application ref in"=w331) -> ("Application ref out"=w330:refnum<vi>)  [unwired: 8 in, 1 out]
            n163 = Write to Binary File(file (use dialog)=w360, data=w355, error in=w348, 5:FALSE ("prepend array or string size? (T)")) -> (refnum out=w359:refnum<file>, error out=w347:errorcluster)  [unwired: 2 in, 1 out]
            n164 = call <userlib>:"Z-Ctrl Setpoint Set.vi"("Z Controller setpoint"=w335, "Application ref in"=w330) -> ("Application ref out"=w337:refnum<vi>)  [unwired: 8 in, 1 out]
            n165 = Increment(x=w345) -> (x+1=w344:i32)
            n166 = Write to Binary File(file (use dialog)=w359, data=w354, error in=w347, 5:FALSE ("prepend array or string size? (T)")) -> (refnum out=w358:refnum<file>, error out=w346:errorcluster)  [unwired: 2 in, 1 out]
          }
        }
        n167 = Get Date/Time In Seconds() -> (seconds since 1Jan1904=w174:timestamp)
        n168 = local read "total Points"() -> (w180:i32)
        n169 = Subtract(x=w174, y=w179) -> (x-y=w178:dbl)
        n170 = Divide(x=w177, y=w180) -> (x/y=w183:dbl)
        n171 = Subtract(x=w180, y=w177) -> (x-y=w175:i32)
        n172 = Divide(x=w178, y=w177) -> (x/y=w176:dbl)
        n173 = Multiply(x=w176, y=w175) -> (x*y=w173:dbl)
        "remaining" <- w173
        n174 = Multiply(x=w183, y=100.0) -> (x*y=→"Progress":dbl)
        n175 = Add(x=w174, y=w173) -> (x+y=→"ETA":timestamp)
      }
      frame "end" {
        n176 = Close File(refnum=w408) -> ()  [unwired: 1 in, 2 out]
        n177 = Close File(refnum=w406) -> (path=w405:path)  [unwired: 1 in, 1 out]
        n178 = local write "Status"("finishing" ("Status")) -> ()
        n179 = call "STSGrid.vi"("Binary Spectroscopy File"=w405) -> ()  [unwired: 11 in]
        n180 = Bundle(w413, w413) -> (w435:cluster{sgl[][], sgl[][]})  [unwired: 1 in]
        n181 = Build Array(w435) -> (w434:cluster{sgl[][], sgl[][]}[])
        n182 = Unbundle By Name(w423) -> ("center X (m)"=w421:sgl, "center Y (m)"=w420:sgl, "angle (deg)"=w419:sgl, "width (m)"=w418:sgl, "height (m)"=w417:sgl)
        n183 = Strip Path(path=w393) -> (stripped path=w427:path, name=w426:string)
        n184 = Get Date/Time In Seconds() -> (seconds since 1Jan1904=w389:timestamp)
        n185 = Bundle By Name(cluster=T5 {"up/down"=FALSE, "time/line"=0.0, "start time"=timestamp(0 s since 1904-01-01), "end time"=timestamp(0 s since 1904-01-01)} ("Scan param"), "up/down"=TRUE, "time/line"=sgl nan ("input 7"), "start time"=w431, "end time"=w389) -> (w430:T5)
        n186 = Bundle By Name(cluster=T3 {"center X"=0.0, "center Y"=0.0, "angle"=0.0, "width"=0.0, "height"=0.0, "# pixels"=0, "# lines"=0} ("Scanfield"), "center X"=w421, "center Y"=w420, "angle"=w419, "width"=w418, "height"=w417, "# lines"=w414, "# pixels"=w415) -> (w416:T3)
        n187 = Bundle("stripped path"=w427, "name"=w426) -> (w425:cluster{"stripped path":path, "name":string})  [unwired: 1 in]
        n188 = call <userlib>:"Save sxm File.vi"("Auto file naming? (T)"=FALSE, "Scanfield"=w416, "Scan param"=w430, "error in (no error)"=w424, "Channels data"=w434, "Channels config"=T4 [{"Name"="Z (m)", "Calibration"=1.0, "Offset"=0.0, "Channel index"=0}], "Filename control"=w425) -> ("error out"=w400:errorcluster)  [unwired: 2 in, 2 out]
        n189 = Strip Path(path=w393) -> (stripped path=w404:path)  [unwired: 1 out]
        n190 = Strip Path(path=w404) -> (stripped path=w403:path)  [unwired: 1 out]
        n191 = call <userlib>:"Get Session Path.vi"("error in (no error)"=w400, "Application ref in"=w399) -> ("error out"=w396:errorcluster, "Session path"=w398:path, "Application ref out"=w382:refnum<vi>)  [unwired: 7 in]
        n192 = Path To String(path=w393) -> (string=w392:string)
        n193 = Path To String(path=w403) -> (string=w401:string)
        n194 = call "SXM.vi"("Path"=w398, "Delete"=FALSE, "error in"=w396) -> ("error out"=w395:errorcluster)  [unwired: 7 in]
        n195 = call "ChangeSessionV2.vi"("error in (no error)"=w395, "Session"=w401) -> ("error out"=w394:errorcluster)
        n196 = Format Date/Time String(time format string (%c)=" Finished at %y%m%d - %H%M%S ", seconds (now)=w389) -> (date/time string=w388:string)  [unwired: 1 in]
        n197 = Concatenate Strings(w392, "\r\n", w388) -> (w391:string)
        n198 = Search and Replace String(input string="Email when finished", search string="@") -> (number of replacements=w384:i32)  [unwired: 6 in, 3 out]
        n199 = Greater Than 0?(x=w384) -> (x > 0?=w383:bool)
        n200 = case shown="True" w383 {
          tunnel: w394 -> [_ w442]
          tunnel: w391 -> [_ w440]
          tunnel: "Email when finished" -> [_ w439]
          frame False {
          }
          frame True {
            n201 = call "Send Email"("error in"=w442, "Message"=w440, "Subject"="Grid Finished", "Recipients"=w439) -> ()  [unwired: 7 in, 1 out]
          }
        }
        n202 = call <userlib>:"BiasSpectroscopy SetProperties.vi"("Application ref in"=w382, "Z-Controller hold (no change)"=enum16{"no change", "on", "off"}."on") -> ("Application ref out"=w380:refnum<vi>)  [unwired: 12 in, 1 out]
        n203 = call <userlib>:"TipLift Set.vi"("TipLift (m)"=sgl 0.0, "Application ref in"=w380) -> ("Application ref out"=w379:refnum<vi>)  [unwired: 8 in, 1 out]
      }
    }
    "Error out" <- w42
    "Points taken" <- w10
    "X Offset" <- w9
    "Y Offset" <- w8
  }
